vi "ClusterWithArrays.vi"(9 "Which Array Elements Are Using Default Values":T1={"Array"=[FALSE, FALSE, FALSE], "Array 2"=[FALSE, FALSE, FALSE], "Array 3"=[FALSE, FALSE, FALSE], "Array 4"=[FALSE, FALSE, FALSE, FALSE]}, 11 "Cluster":T2={"Numeric"=0.0, "Array"=[11.0, 22.0, 44.0], "Array 2"=["One", "Two", "Three"], "Array 3"=[55, 88, 999], "Array 4"=[1.0+2.0i, 3.0+4.0i, 5.0+6.0i, 7.0+8.0i]}) -> (3 "All Default Values Are Equal":bool)   [LabVIEW 2010]
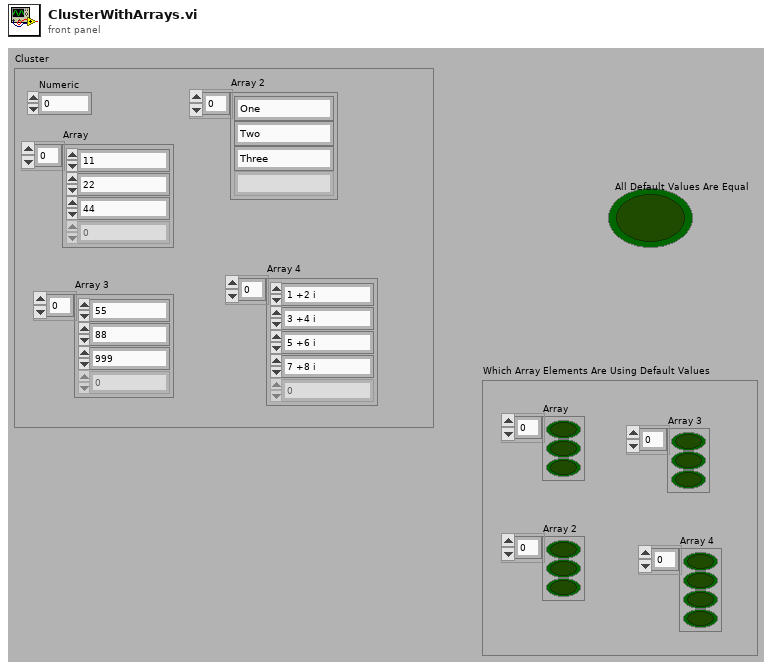
[diagram p1: front panel]
types:
  T1 = cluster{"Array":bool[], "Array 2":bool[], "Array 3":bool[], "Array 4":bool[]}
  T2 = cluster{"Numeric":dbl, "Array":dbl[], "Array 2":string[], "Array 3":i64[], "Array 4":csg[]}
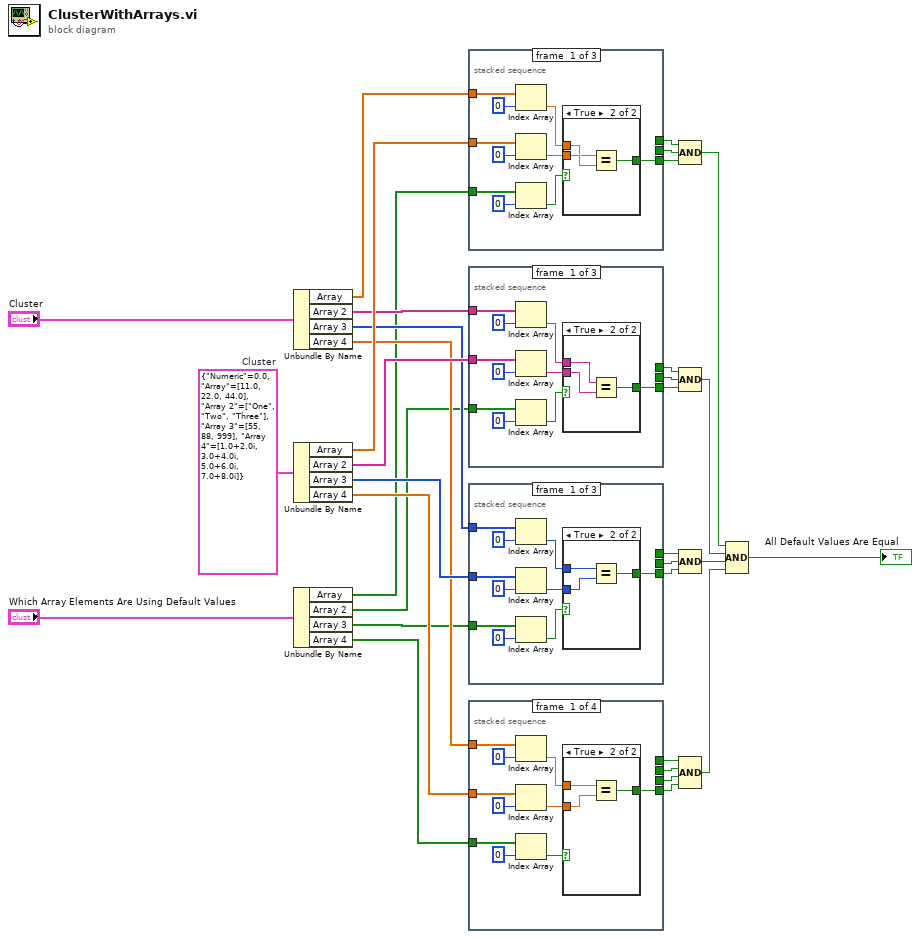
[diagram p0: block diagram]
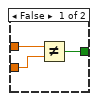
[diagram p2: hidden frame]
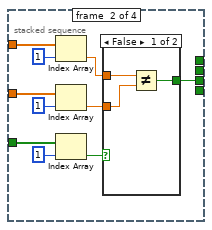
[diagram p3: hidden frame]
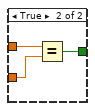
[diagram p4: hidden frame]
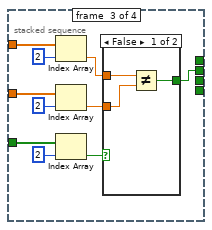
[diagram p5: hidden frame]
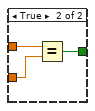
[diagram p6: hidden frame]
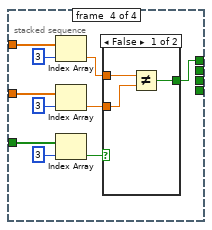
[diagram p7: hidden frame]
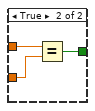
[diagram p8: hidden frame]
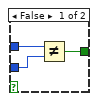
[diagram p9: hidden frame]
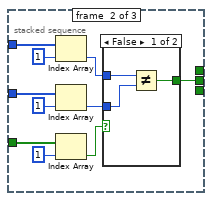
[diagram p10: hidden frame]
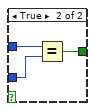
[diagram p11: hidden frame]
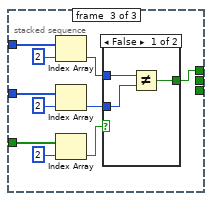
[diagram p12: hidden frame]
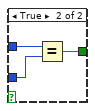
[diagram p13: hidden frame]
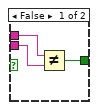
[diagram p14: hidden frame]
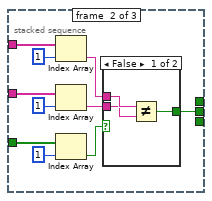
[diagram p15: hidden frame]
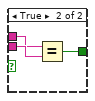
[diagram p16: hidden frame]
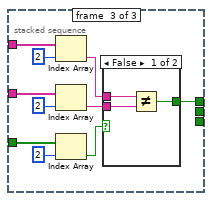
[diagram p17: hidden frame]
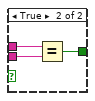
[diagram p18: hidden frame]
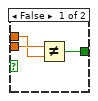
[diagram p19: hidden frame]
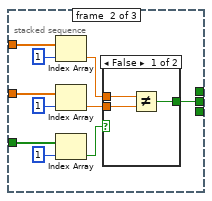
[diagram p20: hidden frame]
diagram:
  w32 = T2 {"Numeric"=0.0, "Array"=[11.0, 22.0, 44.0], "Array 2"=["One", "Two", "Three"], "Array 3"=[55, 88, 999], "Array 4"=[1.0+2.0i, 3.0+4.0i, 5.0+6.0i, 7.0+8.0i]}  # Cluster
  n1 = Unbundle By Name("Cluster") -> ("Array"=w31:dbl[], "Array 2"=w29:string[], "Array 3"=w27:i64[], "Array 4"=w25:csg[])
  n2 = Unbundle By Name(w32) -> ("Array"=w30:dbl[], "Array 2"=w28:string[], "Array 3"=w26:i64[], "Array 4"=w24:csg[])
  n3 = Unbundle By Name("Which Array Elements Are Using Default Values") -> ("Array"=w22:bool[], "Array 2"=w21:bool[], "Array 3"=w20:bool[], "Array 4"=w19:bool[])
  n4 = stacked-sequence {
    tunnel: w22 -> [w43 w51 w67]
    tunnel: w31 -> [w37 w53 w69]
    tunnel: w30 -> [w36 w52 w68]
    tunnel: [w40 _ _] -> w11
    tunnel: [_ w50 _] -> w12
    tunnel: [_ _ w66] -> w13
    frame #0 {
      n5 = Index Array(array=w37, index=0) -> (element=w34:dbl)
      n6 = Index Array(array=w36, index=0) -> (element=w35:dbl)
      n7 = Index Array(array=w43, index=0) -> (element=w42:bool)
      n8 = case shown="True" w42 {
        tunnel: [w44 w49] -> w40
        tunnel: w35 -> [w45 w48]
        tunnel: w34 -> [w46 w47]
        frame False {
          n9 = Not Equal?(x=w46, y=w45) -> (x != y?=w44:bool)
        }
        frame True {
          n10 = Equal?(x=w47, y=w48) -> (x = y?=w49:bool)
        }
      }
    }
    frame #1 {
      n11 = Index Array(array=w53, index=1) -> (element=w54:dbl)
      n12 = Index Array(array=w52, index=1) -> (element=w55:dbl)
      n13 = Index Array(array=w51, index=1) -> (element=w59:bool)
      n14 = case shown="False" w59 {
        tunnel: [w60 w65] -> w50
        tunnel: w55 -> [w61 w64]
        tunnel: w54 -> [w62 w63]
        frame False {
          n15 = Not Equal?(x=w62, y=w61) -> (x != y?=w60:bool)
        }
        frame True {
          n16 = Equal?(x=w63, y=w64) -> (x = y?=w65:bool)
        }
      }
    }
    frame #2 {
      n17 = Index Array(array=w69, index=2) -> (element=w70:dbl)
      n18 = Index Array(array=w68, index=2) -> (element=w71:dbl)
      n19 = Index Array(array=w67, index=2) -> (element=w75:bool)
      n20 = case shown="False" w75 {
        tunnel: [w76 w81] -> w66
        tunnel: w71 -> [w77 w80]
        tunnel: w70 -> [w78 w79]
        frame False {
          n21 = Not Equal?(x=w78, y=w77) -> (x != y?=w76:bool)
        }
        frame True {
          n22 = Equal?(x=w79, y=w80) -> (x = y?=w81:bool)
        }
      }
    }
  }
  n23 = stacked-sequence {
    tunnel: w21 -> [w91 w99 w115]
    tunnel: w29 -> [w85 w101 w117]
    tunnel: w28 -> [w84 w100 w116]
    tunnel: [w88 _ _] -> w8
    tunnel: [_ w98 _] -> w9
    tunnel: [_ _ w114] -> w10
    frame #0 {
      n24 = Index Array(array=w85, index=0) -> (element=w82:string)
      n25 = Index Array(array=w84, index=0) -> (element=w83:string)
      n26 = Index Array(array=w91, index=0) -> (element=w90:bool)
      n27 = case shown="True" w90 {
        tunnel: [w92 w97] -> w88
        tunnel: w83 -> [w93 w96]
        tunnel: w82 -> [w94 w95]
        frame False {
          n28 = Not Equal?(x=w94, y=w93) -> (x != y?=w92:bool)
        }
        frame True {
          n29 = Equal?(x=w95, y=w96) -> (x = y?=w97:bool)
        }
      }
    }
    frame #1 {
      n30 = Index Array(array=w101, index=1) -> (element=w102:string)
      n31 = Index Array(array=w100, index=1) -> (element=w103:string)
      n32 = Index Array(array=w99, index=1) -> (element=w107:bool)
      n33 = case shown="False" w107 {
        tunnel: [w108 w113] -> w98
        tunnel: w103 -> [w109 w112]
        tunnel: w102 -> [w110 w111]
        frame False {
          n34 = Not Equal?(x=w110, y=w109) -> (x != y?=w108:bool)
        }
        frame True {
          n35 = Equal?(x=w111, y=w112) -> (x = y?=w113:bool)
        }
      }
    }
    frame #2 {
      n36 = Index Array(array=w117, index=2) -> (element=w118:string)
      n37 = Index Array(array=w116, index=2) -> (element=w119:string)
      n38 = Index Array(array=w115, index=2) -> (element=w123:bool)
      n39 = case shown="False" w123 {
        tunnel: [w124 w129] -> w114
        tunnel: w119 -> [w125 w128]
        tunnel: w118 -> [w126 w127]
        frame False {
          n40 = Not Equal?(x=w126, y=w125) -> (x != y?=w124:bool)
        }
        frame True {
          n41 = Equal?(x=w127, y=w128) -> (x = y?=w129:bool)
        }
      }
    }
  }
  n42 = stacked-sequence {
    tunnel: w20 -> [w139 w147 w163]
    tunnel: w27 -> [w133 w149 w165]
    tunnel: [w136 _ _] -> w5
    tunnel: [_ w146 _] -> w6
    tunnel: [_ _ w162] -> w7
    tunnel: w26 -> [w130 w148 w164]
    frame #0 {
      n43 = Index Array(array=w133, index=0) -> (element=w131:i64)
      n44 = Index Array(array=w130, index=0) -> (element=w132:i64)
      n45 = Index Array(array=w139, index=0) -> (element=w138:bool)
      n46 = case shown="True" w138 {
        tunnel: [w140 w145] -> w136
        tunnel: w132 -> [w141 w144]
        tunnel: w131 -> [w142 w143]
        frame False {
          n47 = Not Equal?(x=w142, y=w141) -> (x != y?=w140:bool)
        }
        frame True {
          n48 = Equal?(x=w143, y=w144) -> (x = y?=w145:bool)
        }
      }
    }
    frame #1 {
      n49 = Index Array(array=w149, index=1) -> (element=w150:i64)
      n50 = Index Array(array=w148, index=1) -> (element=w151:i64)
      n51 = Index Array(array=w147, index=1) -> (element=w155:bool)
      n52 = case shown="False" w155 {
        tunnel: [w156 w161] -> w146
        tunnel: w151 -> [w157 w160]
        tunnel: w150 -> [w158 w159]
        frame False {
          n53 = Not Equal?(x=w158, y=w157) -> (x != y?=w156:bool)
        }
        frame True {
          n54 = Equal?(x=w159, y=w160) -> (x = y?=w161:bool)
        }
      }
    }
    frame #2 {
      n55 = Index Array(array=w165, index=2) -> (element=w166:i64)
      n56 = Index Array(array=w164, index=2) -> (element=w167:i64)
      n57 = Index Array(array=w163, index=2) -> (element=w171:bool)
      n58 = case shown="False" w171 {
        tunnel: [w172 w177] -> w162
        tunnel: w167 -> [w173 w176]
        tunnel: w166 -> [w174 w175]
        frame False {
          n59 = Not Equal?(x=w174, y=w173) -> (x != y?=w172:bool)
        }
        frame True {
          n60 = Equal?(x=w175, y=w176) -> (x = y?=w177:bool)
        }
      }
    }
  }
  n61 = stacked-sequence {
    tunnel: w19 -> [w187 w195 w211 w227]
    tunnel: w25 -> [w181 w197 w213 w229]
    tunnel: w24 -> [w180 w196 w212 w228]
    tunnel: [w184 _ _ _] -> w2
    tunnel: [_ w194 _ _] -> w3
    tunnel: [_ _ w210 _] -> w4
    tunnel: [_ _ _ w226] -> w1
    frame #0 {
      n62 = Index Array(array=w181, index=0) -> (element=w178:csg)
      n63 = Index Array(array=w180, index=0) -> (element=w179:csg)
      n64 = Index Array(array=w187, index=0) -> (element=w186:bool)
      n65 = case shown="True" w186 {
        tunnel: [w188 w193] -> w184
        tunnel: w179 -> [w189 w192]
        tunnel: w178 -> [w190 w191]
        frame False {
          n66 = Not Equal?(x=w190, y=w189) -> (x != y?=w188:bool)
        }
        frame True {
          n67 = Equal?(x=w191, y=w192) -> (x = y?=w193:bool)
        }
      }
    }
    frame #1 {
      n68 = Index Array(array=w197, index=1) -> (element=w198:csg)
      n69 = Index Array(array=w196, index=1) -> (element=w199:csg)
      n70 = Index Array(array=w195, index=1) -> (element=w203:bool)
      n71 = case shown="False" w203 {
        tunnel: [w204 w209] -> w194
        tunnel: w199 -> [w205 w208]
        tunnel: w198 -> [w206 w207]
        frame False {
          n72 = Not Equal?(x=w206, y=w205) -> (x != y?=w204:bool)
        }
        frame True {
          n73 = Equal?(x=w207, y=w208) -> (x = y?=w209:bool)
        }
      }
    }
    frame #2 {
      n74 = Index Array(array=w213, index=2) -> (element=w214:csg)
      n75 = Index Array(array=w212, index=2) -> (element=w215:csg)
      n76 = Index Array(array=w211, index=2) -> (element=w219:bool)
      n77 = case shown="False" w219 {
        tunnel: [w220 w225] -> w210
        tunnel: w215 -> [w221 w224]
        tunnel: w214 -> [w222 w223]
        frame False {
          n78 = Not Equal?(x=w222, y=w221) -> (x != y?=w220:bool)
        }
        frame True {
          n79 = Equal?(x=w223, y=w224) -> (x = y?=w225:bool)
        }
      }
    }
    frame #3 {
      n80 = Index Array(array=w229, index=3) -> (element=w230:csg)
      n81 = Index Array(array=w228, index=3) -> (element=w231:csg)
      n82 = Index Array(array=w227, index=3) -> (element=w235:bool)
      n83 = case shown="False" w235 {
        tunnel: [w236 w241] -> w226
        tunnel: w231 -> [w237 w240]
        tunnel: w230 -> [w238 w239]
        frame False {
          n84 = Not Equal?(x=w238, y=w237) -> (x != y?=w236:bool)
        }
        frame True {
          n85 = Equal?(x=w239, y=w240) -> (x = y?=w241:bool)
        }
      }
    }
  }
  n86 = Compound Arithmetic op=AND(w13, w12, w11) -> (w18:bool)
  n87 = Compound Arithmetic op=AND(w10, w9, w8) -> (w17:bool)
  n88 = Compound Arithmetic op=AND(w7, w6, w5) -> (w16:bool)
  n89 = Compound Arithmetic op=AND(w1, w4, w3, w2) -> (w15:bool)
  n90 = Compound Arithmetic op=AND(w18, w17, w16, w15) -> (→"All Default Values Are Equal":bool)
